vi "ACTION.vi"(8 "error in (no error)":errorcluster, 9 "STEP State":T1, 10 "CORE":refnum<queue>, 11 "AutoZero in":refnum<class "AutoZero.lvclass">) -> (0 "error out":errorcluster, 3 "AutoZero out":refnum<class "AutoZero.lvclass">)   [LabVIEW 2014, in "SeqLoop.lvlib" / "STEP Classes.lvlib" / "AutoZero.lvclass"]
uses:
  AutoZero.lvclass
  TypeDefs/STEP State.ctl
  APIs/Message Queue/Message Cluster.ctl
  AutoZero.lvclass/AutoZero.ctl
  APIs/Message Queue/Enqueue Message (Array).vi
  APIs/Message Queue/Enqueue Message (Single).vi
  APIs/Message Queue/WINFAS 2 Message Queue.lvlib
  SeqLoop.lvlib
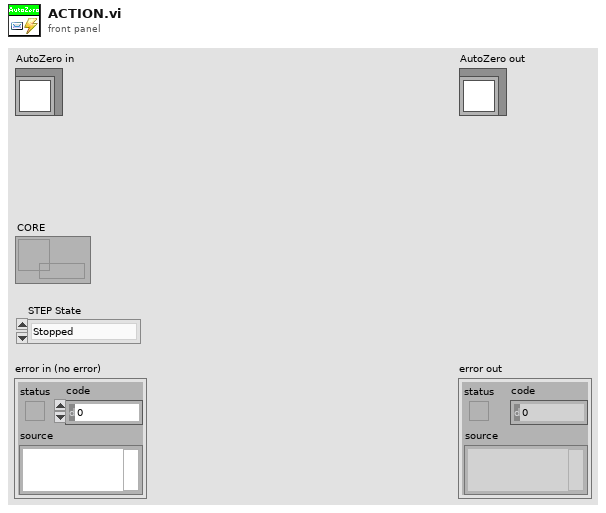
[diagram p1: front panel]
types:
  T1 = typedef "SeqLoop.lvlib/STEP State.ctl" = enum16{"Stopped", "First Call", "Idle...", "Advance OK", "Alarm", "Output Security", "Error"}
  T2 = cluster{"HWSync 1":bool, "HWSync 2":bool, "HWSync 3":bool, "HWSync 4":bool, "HWSync 5":bool}
  T3 = cluster{"HWAsync 1":bool, "HWAsync 2":bool, "HWAsync 3":bool, "HWAsync 4":bool, "HWAsync 5":bool, "HWAsync 6":bool, "HWAsync 7":bool, "HWAsync 8":bool, "HWAsync 9":bool, "HWAsync 10":bool}
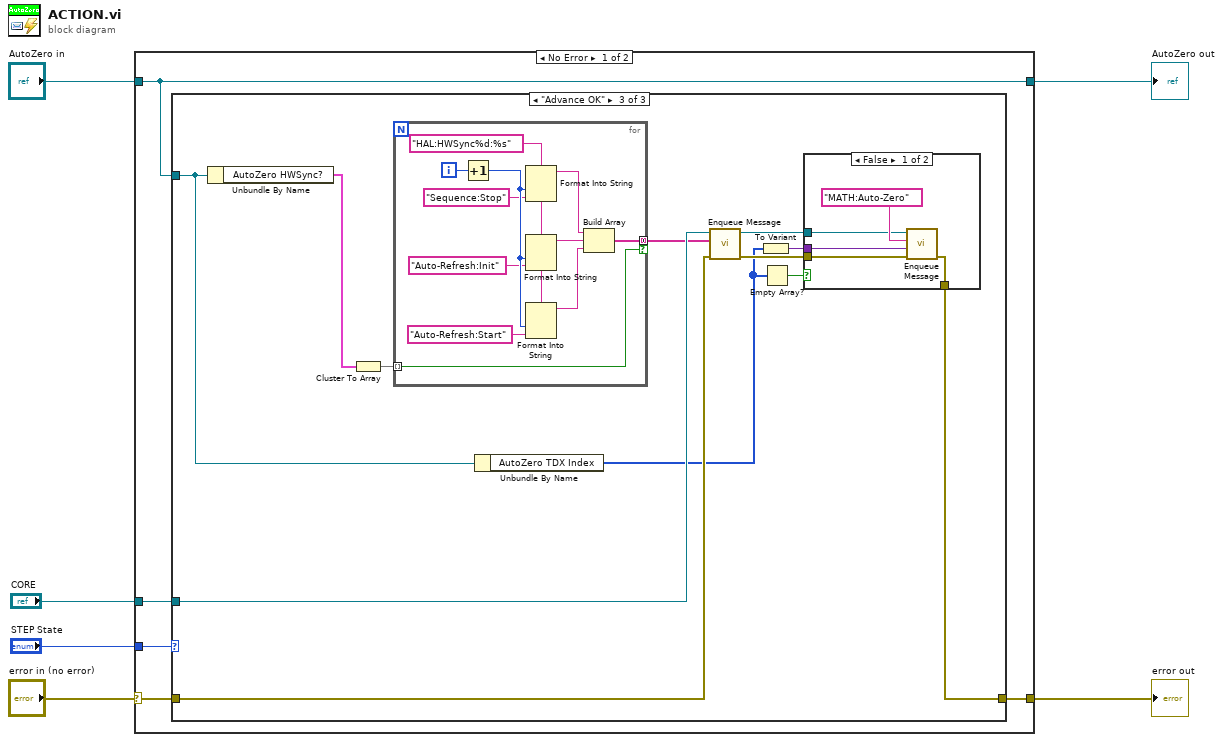
[diagram p0: block diagram]
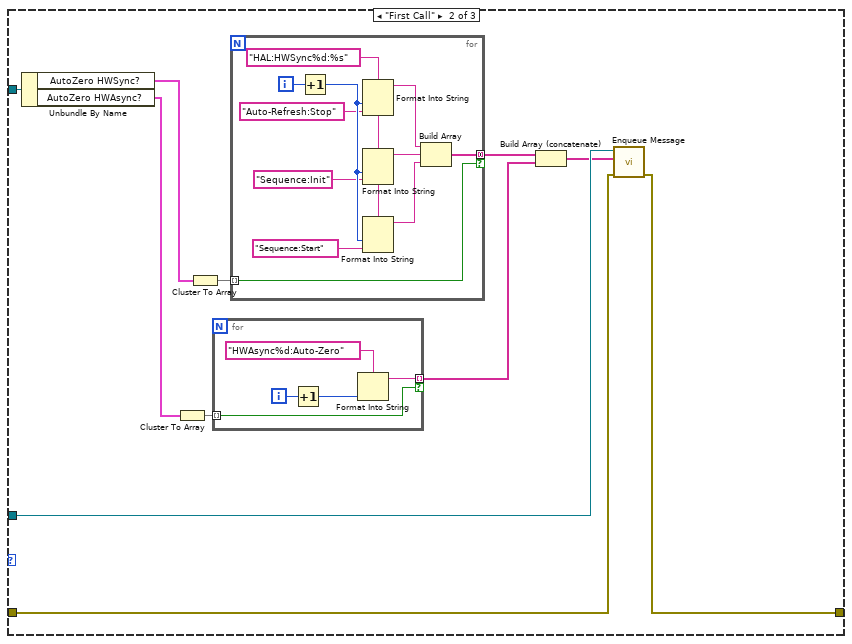
[diagram p3: hidden frame]
diagram:
  n1 = case shown="No Error" "error in (no error)" {
    selector: "error in (no error)" -> [w8 w70]
    tunnel: [w7 w70] -> w3
    tunnel: [w9 w69] -> w5
    tunnel: "AutoZero in" -> [w9 w69]
    tunnel: "CORE" -> [w10 _]
    tunnel: "STEP State" -> [w11 _]
    frame No Error {
      n2 = case shown="\"Advance OK\"" w11 {
        tunnel: w10 -> [_ w16 w49]
        tunnel: w9 -> [_ w22 w44]
        tunnel: w8 -> [w12 w14 w48]
        tunnel: [w12 w13 w45] -> w7
        frame Default {
        }
        frame "First Call" {
          n3 = Unbundle By Name(w22) -> ("AutoZero HWSync?"=w21:T2, "AutoZero HWAsync?"=w20:T3)
          n4 = Cluster To Array(cluster=w20) -> (array=w19:bool[])
          n5 = Cluster To Array(cluster=w21) -> (array=w23:bool[])
          n6 = for {
            tunnel: w19 -> [w24] mode=indexing
            tunnel: [w25] -> w17 mode=indexing if=w24
            i -> [w27]
            n7 = Increment(x=w27) -> (x+1=w26:i32)
            n8 = Format Into String(format string="HWAsync%d:Auto-Zero", w26) -> (resulting string=w25:string)  [unwired: 2 in, 1 out]
          }
          n9 = for {
            tunnel: w23 -> [w29] mode=indexing
            tunnel: [w30] -> w18 mode=concatenating if=w29
            i -> [w39]
            w38 = "HAL:HWSync%d:%s" ("format string")
            n10 = Increment(x=w39) -> (x+1=w37:i32)
            n11 = Format Into String(format string=w38, w37, "Auto-Refresh:Stop" ("format string")) -> (resulting string=w33:string)  [unwired: 2 in, 1 out]
            n12 = Format Into String(format string=w38, w37, "Sequence:Init" ("format string")) -> (resulting string=w32:string)  [unwired: 2 in, 1 out]
            n13 = Format Into String(format string=w38, w37, "Sequence:Start" ("format string")) -> (resulting string=w31:string)  [unwired: 2 in, 1 out]
            n14 = Build Array(w33, w32, w31) -> (w30:string[])
          }
          n15 = Build Array (concatenate)(w18, w17) -> (w15:string[])
          n16 = call-poly "Enqueue Message.vi"("error in (no error)"=w14, "Message Array"=w15, "Message Queue"=w16) -> ("error out"=w13:errorcluster)  [unwired: 7 in, 1 out]
        }
        frame "Advance OK" {
          n17 = Unbundle By Name(w44) -> ("AutoZero HWSync?"=w50:T2)
          n18 = Cluster To Array(cluster=w50) -> (array=w51:bool[])
          n19 = for {
            tunnel: w51 -> [w58] mode=indexing
            tunnel: [w59] -> w47 mode=concatenating if=w58
            i -> [w68]
            w67 = "HAL:HWSync%d:%s" ("format string")
            n20 = Increment(x=w68) -> (x+1=w66:i32)
            n21 = Format Into String(format string=w67, w66, "Sequence:Stop" ("format string")) -> (resulting string=w62:string)  [unwired: 2 in, 1 out]
            n22 = Format Into String(format string=w67, w66, "Auto-Refresh:Init" ("format string")) -> (resulting string=w61:string)  [unwired: 2 in, 1 out]
            n23 = Format Into String(format string=w67, w66, "Auto-Refresh:Start" ("format string")) -> (resulting string=w60:string)  [unwired: 2 in, 1 out]
            n24 = Build Array(w62, w61, w60) -> (w59:string[])
          }
          n25 = Unbundle By Name(w44) -> ("AutoZero TDX Index"=w41:i32[])
          n26 = call-poly "Enqueue Message.vi"("error in (no error)"=w48, "Message Array"=w47, "Message Queue"=w49) -> ("error out"=w46:errorcluster, "dup Message Queue"=w43:refnum<queue>)  [unwired: 7 in]
          n27 = To Variant(anything=w41) -> (Variant=w42:variant)
          n28 = Empty Array?(array=w41) -> (empty?=w40:bool)
          n29 = case shown="False" w40 {
            tunnel: w46 -> [w56 w57]
            tunnel: [w55 w57] -> w45
            tunnel: w43 -> [w53 _]
            tunnel: w42 -> [w52 _]
            frame False {
              n30 = call-poly "Enqueue Message.vi"("error in (no error)"=w56, "Message Data"=w52, "Message"="MATH:Auto-Zero" ("format string"), "Message Queue"=w53) -> ("error out"=w55:errorcluster)  [unwired: 6 in, 1 out]
            }
            frame True {
            }
          }
        }
      }
    }
    frame Error {
    }
  }
  "error out" <- w3
  "AutoZero out" <- w5
